vi "LoadVIlocations.vi"(11 "configuration file path":path) -> (0 "error out":errorcluster, 2 "NamesAndLocnsArray":T1[](array[typedef]))   [LabVIEW 2022 SP3]
uses:
  Anemometry Sub Vis/Controls/VInameSizePath.ctl
  <vilib>/Utility/miscctls.llb/LVRectTypeDef.ctl
  <vilib>/Utility/config.llb/Read Key (I32).vi
  <vilib>/Utility/config.llb/Read Key (Path).vi
  <vilib>/Utility/config.llb/NI_LVConfig.lvlib
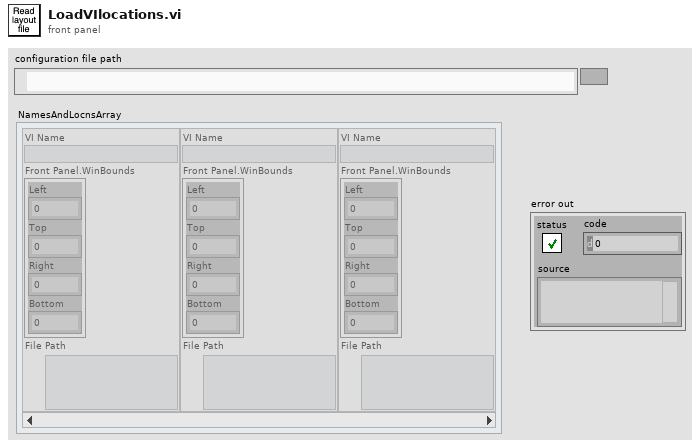
[diagram p1: front panel]
types:
  T1 = typedef "VInameSizePath.ctl" = cluster{"VI Name":string, "Front Panel.WinBounds":T2, "File Path":path}
  T2 = typedef "LVRectTypeDef.ctl" = cluster{"Left":i16, "Top":i16, "Right":i16, "Bottom":i16}
  T3 = typedef "NI_LVConfig.lvlib/Config Data RefNum.ctl" = refnum<k1>
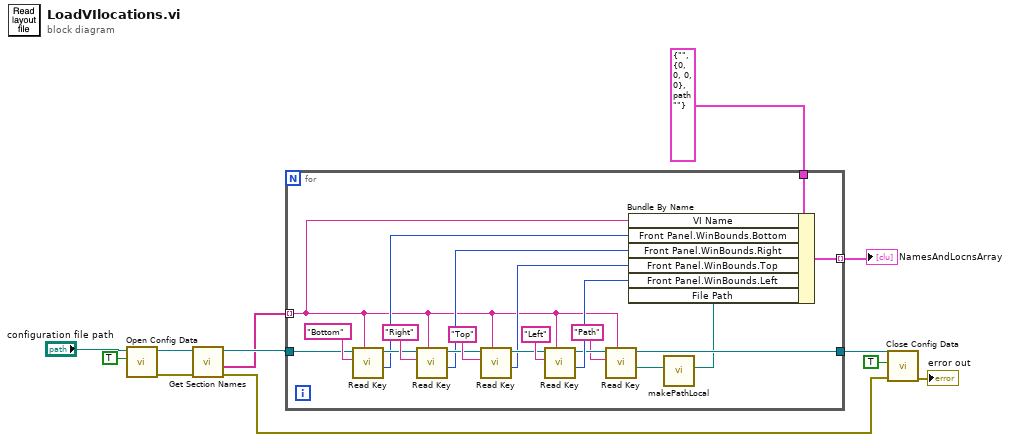
[diagram p0: block diagram]
diagram:
  n1 = call <vilib>:"Open Config Data.vi"("create file if necessary (T)"=TRUE, "configuration file path"="configuration file path") -> ("error out"=w8:errorcluster, "refnum"=w7:T3)  [unwired: 7 in, 1 out]
  n2 = call <vilib>:"Get Section Names.vi"("error in (no error)"=w8, "refnum"=w7) -> ("error out"=w2:errorcluster, "section names"=w5:string[], "refnum out"=w6:T3)  [unwired: 7 in]
  n3 = for {
    tunnel: w6 -> [w28]
    tunnel: [w15] -> w12
    tunnel: w5 -> [w17] mode=indexing
    tunnel: T1 {"VI Name"="", "Front Panel.WinBounds"={"Left"=0, "Top"=0, "Right"=0, "Bottom"=0}, "File Path"=path ""} ("Cluster") -> [w24]
    tunnel: [w19] -> w3 mode=indexing
    n4 = call-poly <vilib>:"Read Key.vi"("section"=w17, "key"="Bottom", "refnum"=w28) -> ("value"=w23:i32, "refnum out"=w27:T3)  [unwired: 5 in, 2 out]
    n5 = call-poly <vilib>:"Read Key.vi"("section"=w17, "key"="Right", "refnum"=w27) -> ("value"=w22:i32, "refnum out"=w26:T3)  [unwired: 5 in, 2 out]
    n6 = call-poly <vilib>:"Read Key.vi"("section"=w17, "key"="Top", "refnum"=w26) -> ("value"=w21:i32, "refnum out"=w25:T3)  [unwired: 5 in, 2 out]
    n7 = call-poly <vilib>:"Read Key.vi"("section"=w17, "key"="Left", "refnum"=w25) -> ("value"=w20:i32, "refnum out"=w18:T3)  [unwired: 5 in, 2 out]
    n8 = call-poly <vilib>:"Read Key.vi"("section"=w17, "key"="Path", "refnum"=w18) -> ("value"=w14:path, "refnum out"=w15:T3)  [unwired: 5 in, 2 out]
    n9 = call "makePathLocal.vi"("storedPath"=w14) -> ("loadPath"=w13:path)  [unwired: 10 in]
    n10 = Bundle By Name(cluster=w24, "VI Name"=w17, "Front Panel.WinBounds.Bottom"=w23, "Front Panel.WinBounds.Right"=w22, "Front Panel.WinBounds.Top"=w21, "Front Panel.WinBounds.Left"=w20, "File Path"=w13) -> (w19:T1)
  }
  "NamesAndLocnsArray" <- w3
  n11 = call <vilib>:"Close Config Data.vi"("error in (no error)"=w2, "write file if changed (T)"=TRUE, "refnum"=w12) -> ("error out"=→"error out":errorcluster)  [unwired: 7 in, 1 out]
